vi "AtlasWavelengths.vi"() -> (0 "error out":errorcluster, 2 "AtlasStat":string[](array[string]), 3 "Wavelengths":dbl[](array[numeric]), 11 "Laser status":bool[](array[boolean]))   [LabVIEW 2019]
uses:
  <vilib>/regexp/Match Regular Expression.xnode
panel:
  out "body":string
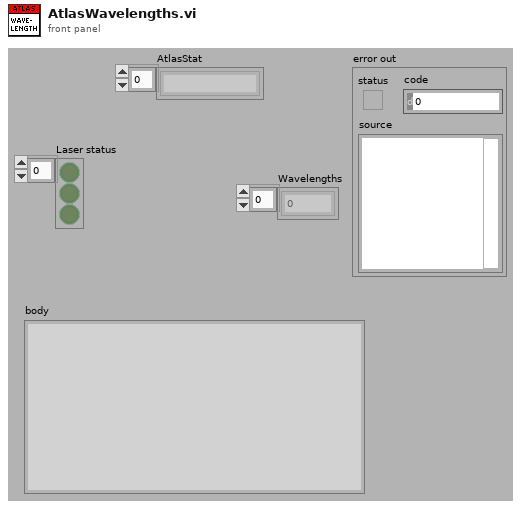
[diagram p1: front panel]
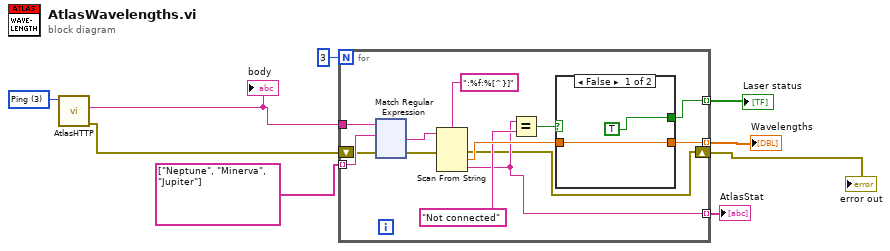
[diagram p0: block diagram]
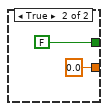
[diagram p2: hidden frame]
diagram:
  w9 = u16 3 items=["Login", "Logout", "get_laser_names", "Ping", "Unlock", "Lock171", "Lock174", "Connect", "Disconnect"] ("Command")
  n1 = call "AtlasHTTP.vi"("Command"=w9) -> ("error out"=w2:errorcluster, "body"=w6:string)  [unwired: 7 in]
  "body" <- w6
  n2 = for {
    N: 3 -> [_]
    tunnel: w6 -> [w22]
    tunnel: string[] ["Neptune", "Minerva", "Jupiter"] -> [w19] mode=indexing
    tunnel: [w17] -> w5 mode=indexing
    tunnel: [w13] -> w4 mode=indexing
    tunnel: [w12] -> w3 mode=indexing
    shift-right: [w10] -> w1
    shift-left: w2 -> [w11]
    n3 = xnode "Match Regular Expression"("input string"=w22, "regular expression"=w19, "error in"=w11) -> ("after match"=w21:string, "error out"=w16:errorcluster)  [unwired: 3 in, 3 out]
    n4 = Scan From String(format string=":%f:%[^}]", input string=w21, error in=w16) -> (error out=w10:errorcluster, output 1=w18:dbl, output 2=w12:string)  [unwired: 3 in, 2 out]
    n5 = Equal?(x=w12, y="Not connected") -> (x = y?=w14:bool)
    n6 = case shown="False" w14 {
      tunnel: w18 -> [w24 _]
      tunnel: [w24 0.0] -> w17
      tunnel: [TRUE FALSE] -> w13
      frame False {
      }
      frame True {
      }
    }
  }
  "Laser status" <- w4
  "Wavelengths" <- w5
  "AtlasStat" <- w3
  "error out" <- w1
